vi "SingleMoleFinder.vi"(6 "Image Src":T1, 7 "error in":errorcluster, 18 "Min Radius (CircleDetection)":sgl=15.0, 19 "Max Radius (CircleDetection)":sgl=50.0, 21 "Keep/Remove Particles (Particle Filter 1)":bool=TRUE, 23 "Selection Values (Particle Filter 1)":T3(array[cluster])=[{"Measurement Parameter"=1, "Range Lower Value"=0.0, "Range Upper Value"=0.0, "Range"=FALSE, "Measurement Type"=FALSE}, {"Measurement Parameter"=0, "Range Lower Value"=15.0, "Range Upper Value"=100.0, "Range"=FALSE, "Measurement Type"=FALSE}] {"Measurement Parameter" items=["Center of Mass X", "Center of Mass Y", "First Pixel X", "First Pixel Y", "Bounding Rect Left", "Bounding Rect Top", "Bounding Rect Right", "Bounding Rect Bottom", "Max Feret Diameter Start X", "Max Feret Diameter Start Y", "Max Feret Diameter End X", "Max Feret Diameter End Y", "Max Horiz. Segment Length Left", "Max Horiz. Segment Length Right", "Max Horiz. Segment Length Row", "-", "Bounding Rect Width", "Bounding Rect Height", "Bounding Rect Diagonal", "Perimeter", "Convex Hull Perimeter", "Holes' Perimeter", "Max Feret Diameter", "Equivalent Ellipse Major Axis", "Equivalent Ellipse Minor Axis", "Equivalent Ellipse Minor Axis (Feret)", "Equivalent Rect Long Side", "Equivalent Rect Short Side", "Equivalent Rect Diagonal", "Equivalent Rect Short Side (Feret)", "Average Horiz. Segment Length", "Average Vert. Segment Length", "Hydraulic Radius", "Waddel Disk Diameter", "-", "Area", "Holes' Area", "Particle & Holes' Area", "Convex Hull Area", "Image Area", "-", "Number of Holes", "Number of Horiz. Segments", "Number of Vert. Segments", "-", "Orientation", "Max Feret Diameter Orientation", "-", "% Area/Image Area", "% Area/(Particle & Holes' Area)", "Ratio of Equivalent Ellipse Axes", "Ratio of Equivalent Rect Sides", "-", "Elongation Factor", "Compactness Factor", "Heywood Circularity Factor", "Type Factor", "-", "Sum X", "Sum Y", "Sum XX", "Sum XY", "Sum YY", "Sum XXX", "Sum XXY", "Sum XYY", "Sum YYY", "-", "Moment of Inertia XX", "Moment of Inertia XY", "Moment of Inertia YY", "Moment of Inertia XXX", "Moment of Inertia XXY", "Moment of Inertia XYY", "Moment of Inertia YYY", "Norm. Moment of Inertia XX", "Norm. Moment of Inertia XY", "Norm. Moment of Inertia YY", "Norm. Moment of Inertia XXX", "Norm. Moment of Inertia XXY", "Norm. Moment of Inertia XYY", "Norm. Moment of Inertia YYY", "Hu Moment 1", "Hu Moment 2", "Hu Moment 3", "Hu Moment 4", "Hu Moment 5", "Hu Moment 6", "Hu Moment 7"]}) -> (15 "Image Out":T1(plugin-control), 20 "Nb Circles (CircleDetection)":i32, 26 "Circles Data (CircleDetection)":T2(array[cluster]), 27 "error out":errorcluster)   [LabVIEW 2011]
uses:
  <vilib>/vision/Image Controls.llb/IMAQ Image.ctl
  <vilib>/vision/NI_Vision_Development_Module.lvlib
panel:
  out "Image Out 10":T1(plugin-control)
  out "Image Out 9":T1(plugin-control)
  out "Image Out 8":T1(plugin-control)
  out "Image Out 7":T1(plugin-control)
  out "Image Out 6":T1(plugin-control)
  out "Image Out 5":T1(plugin-control)
  out "Image Out 4":T1(plugin-control)
  out "Image Out 3":T1(plugin-control)
  out "Image Out 2":T1(plugin-control)
  out "Circles Data (calibrated)":T2(array[cluster])
  out "Number of Particles 2":i32
  out "Number of Particles":i32
  out "Particle Measurements (Pixels)":dbl[][](array[numeric]) format="%.2f"
  out "Particle Measurements (Real-World)":dbl[][](array[numeric]) format="%.2f"
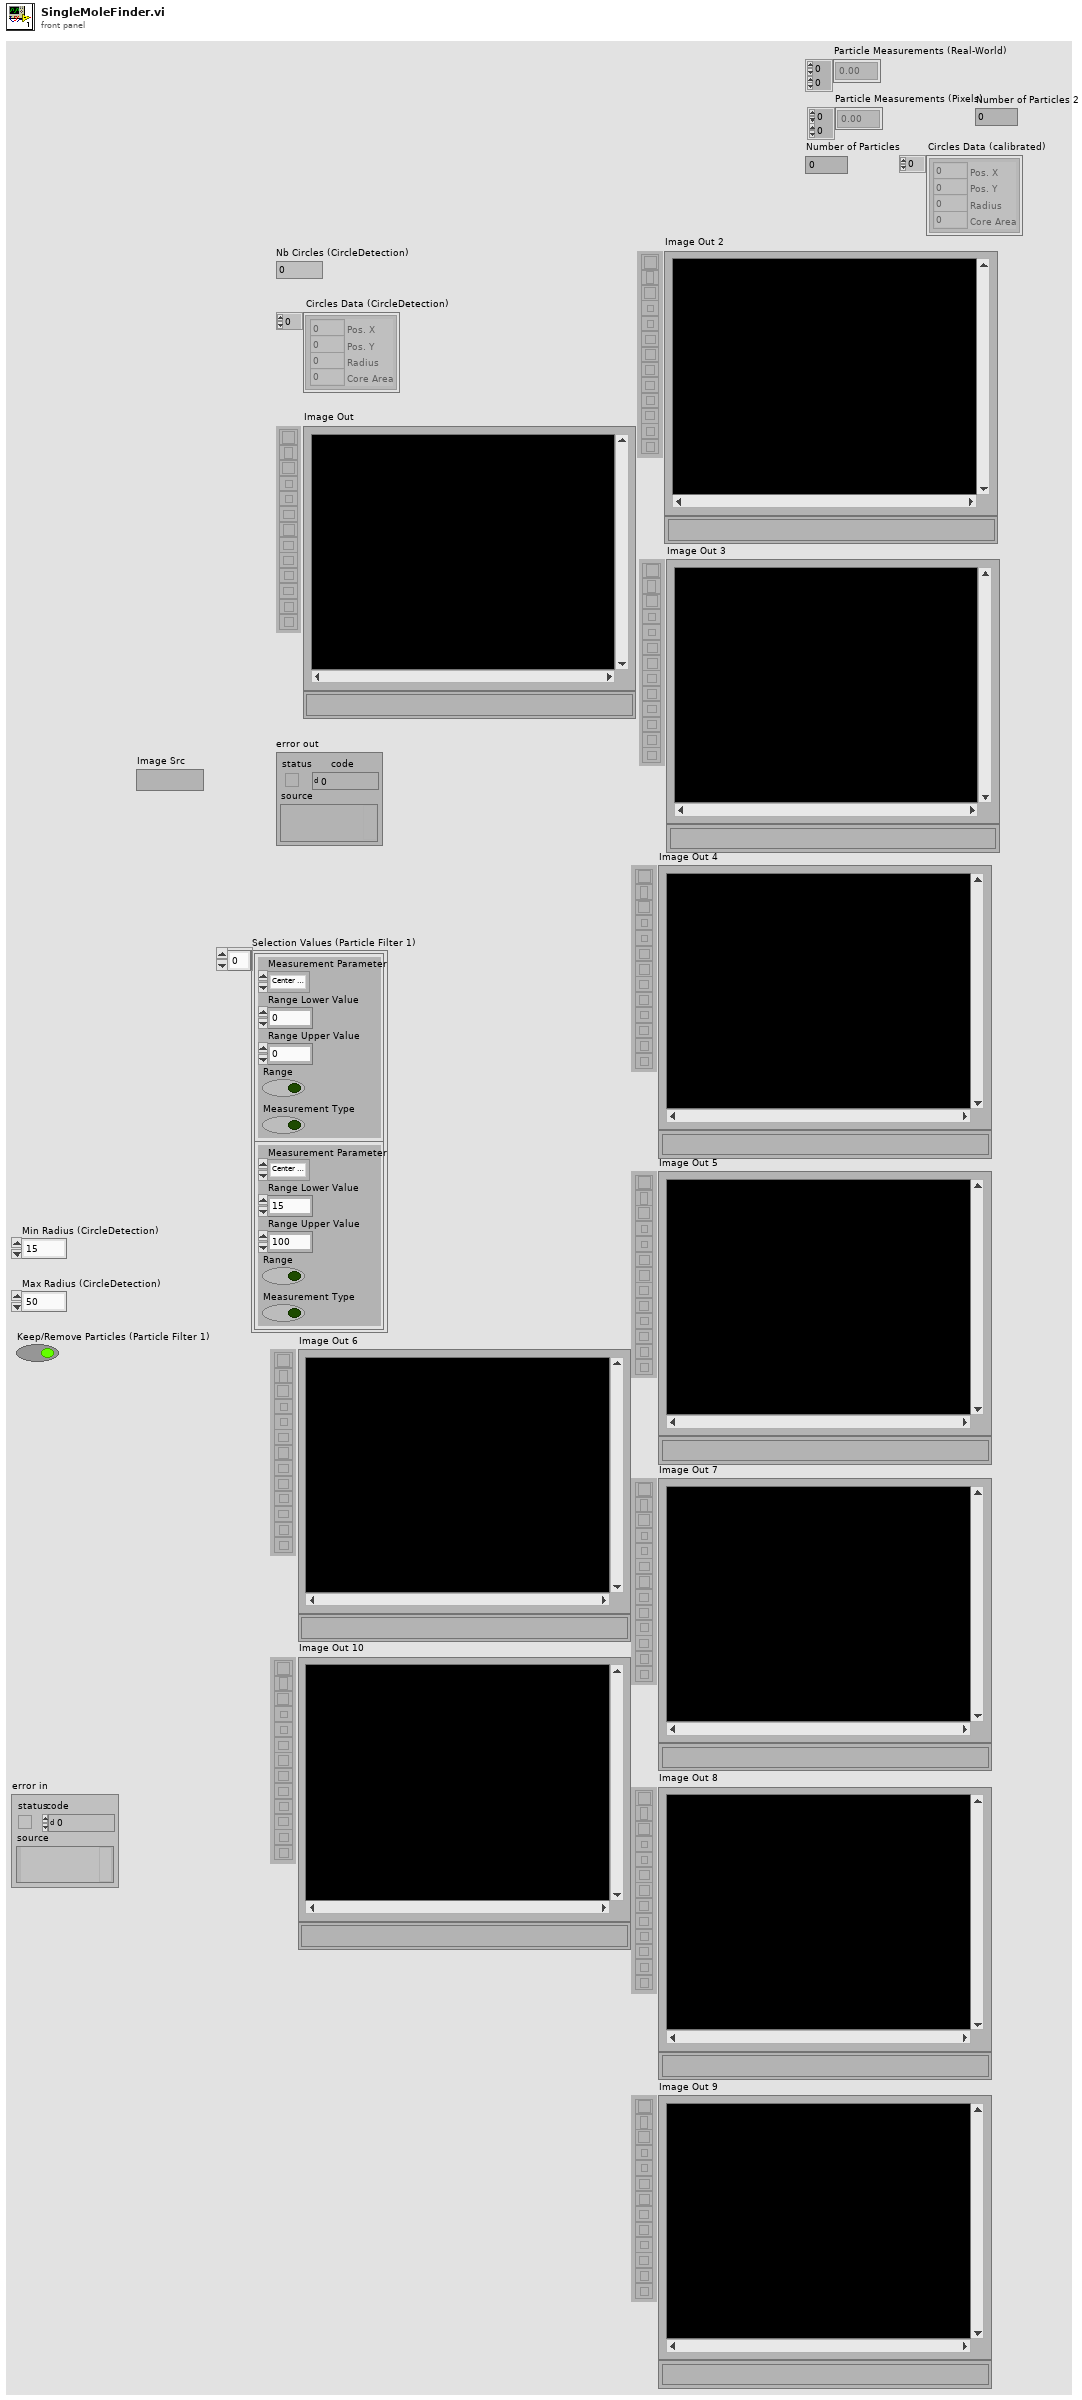
[diagram p1: front panel]
types:
  T1 = typedef "IMAQ Image.ctl" = refnum<image>
  T2 = cluster{"Pos. X":i32, "Pos. Y":i32, "Radius":i32, "Core Area":i32}[]
  T3 = cluster{"Measurement Parameter":i32, "Range Lower Value":dbl, "Range Upper Value":dbl, "Range":bool, "Measurement Type":bool}[]
  T4 = enum32{"AutoM", "Close", "Dilate", "Erode", "Gradient", "Gradient out", "Gradient in", "Hit miss", "Open", "PClose", "POpen", "Thick", "Thin"}
  T5 = enum32{"Linear", "Log", "Exp", "Square", "Square root", "Power X", "Power 1/X"}
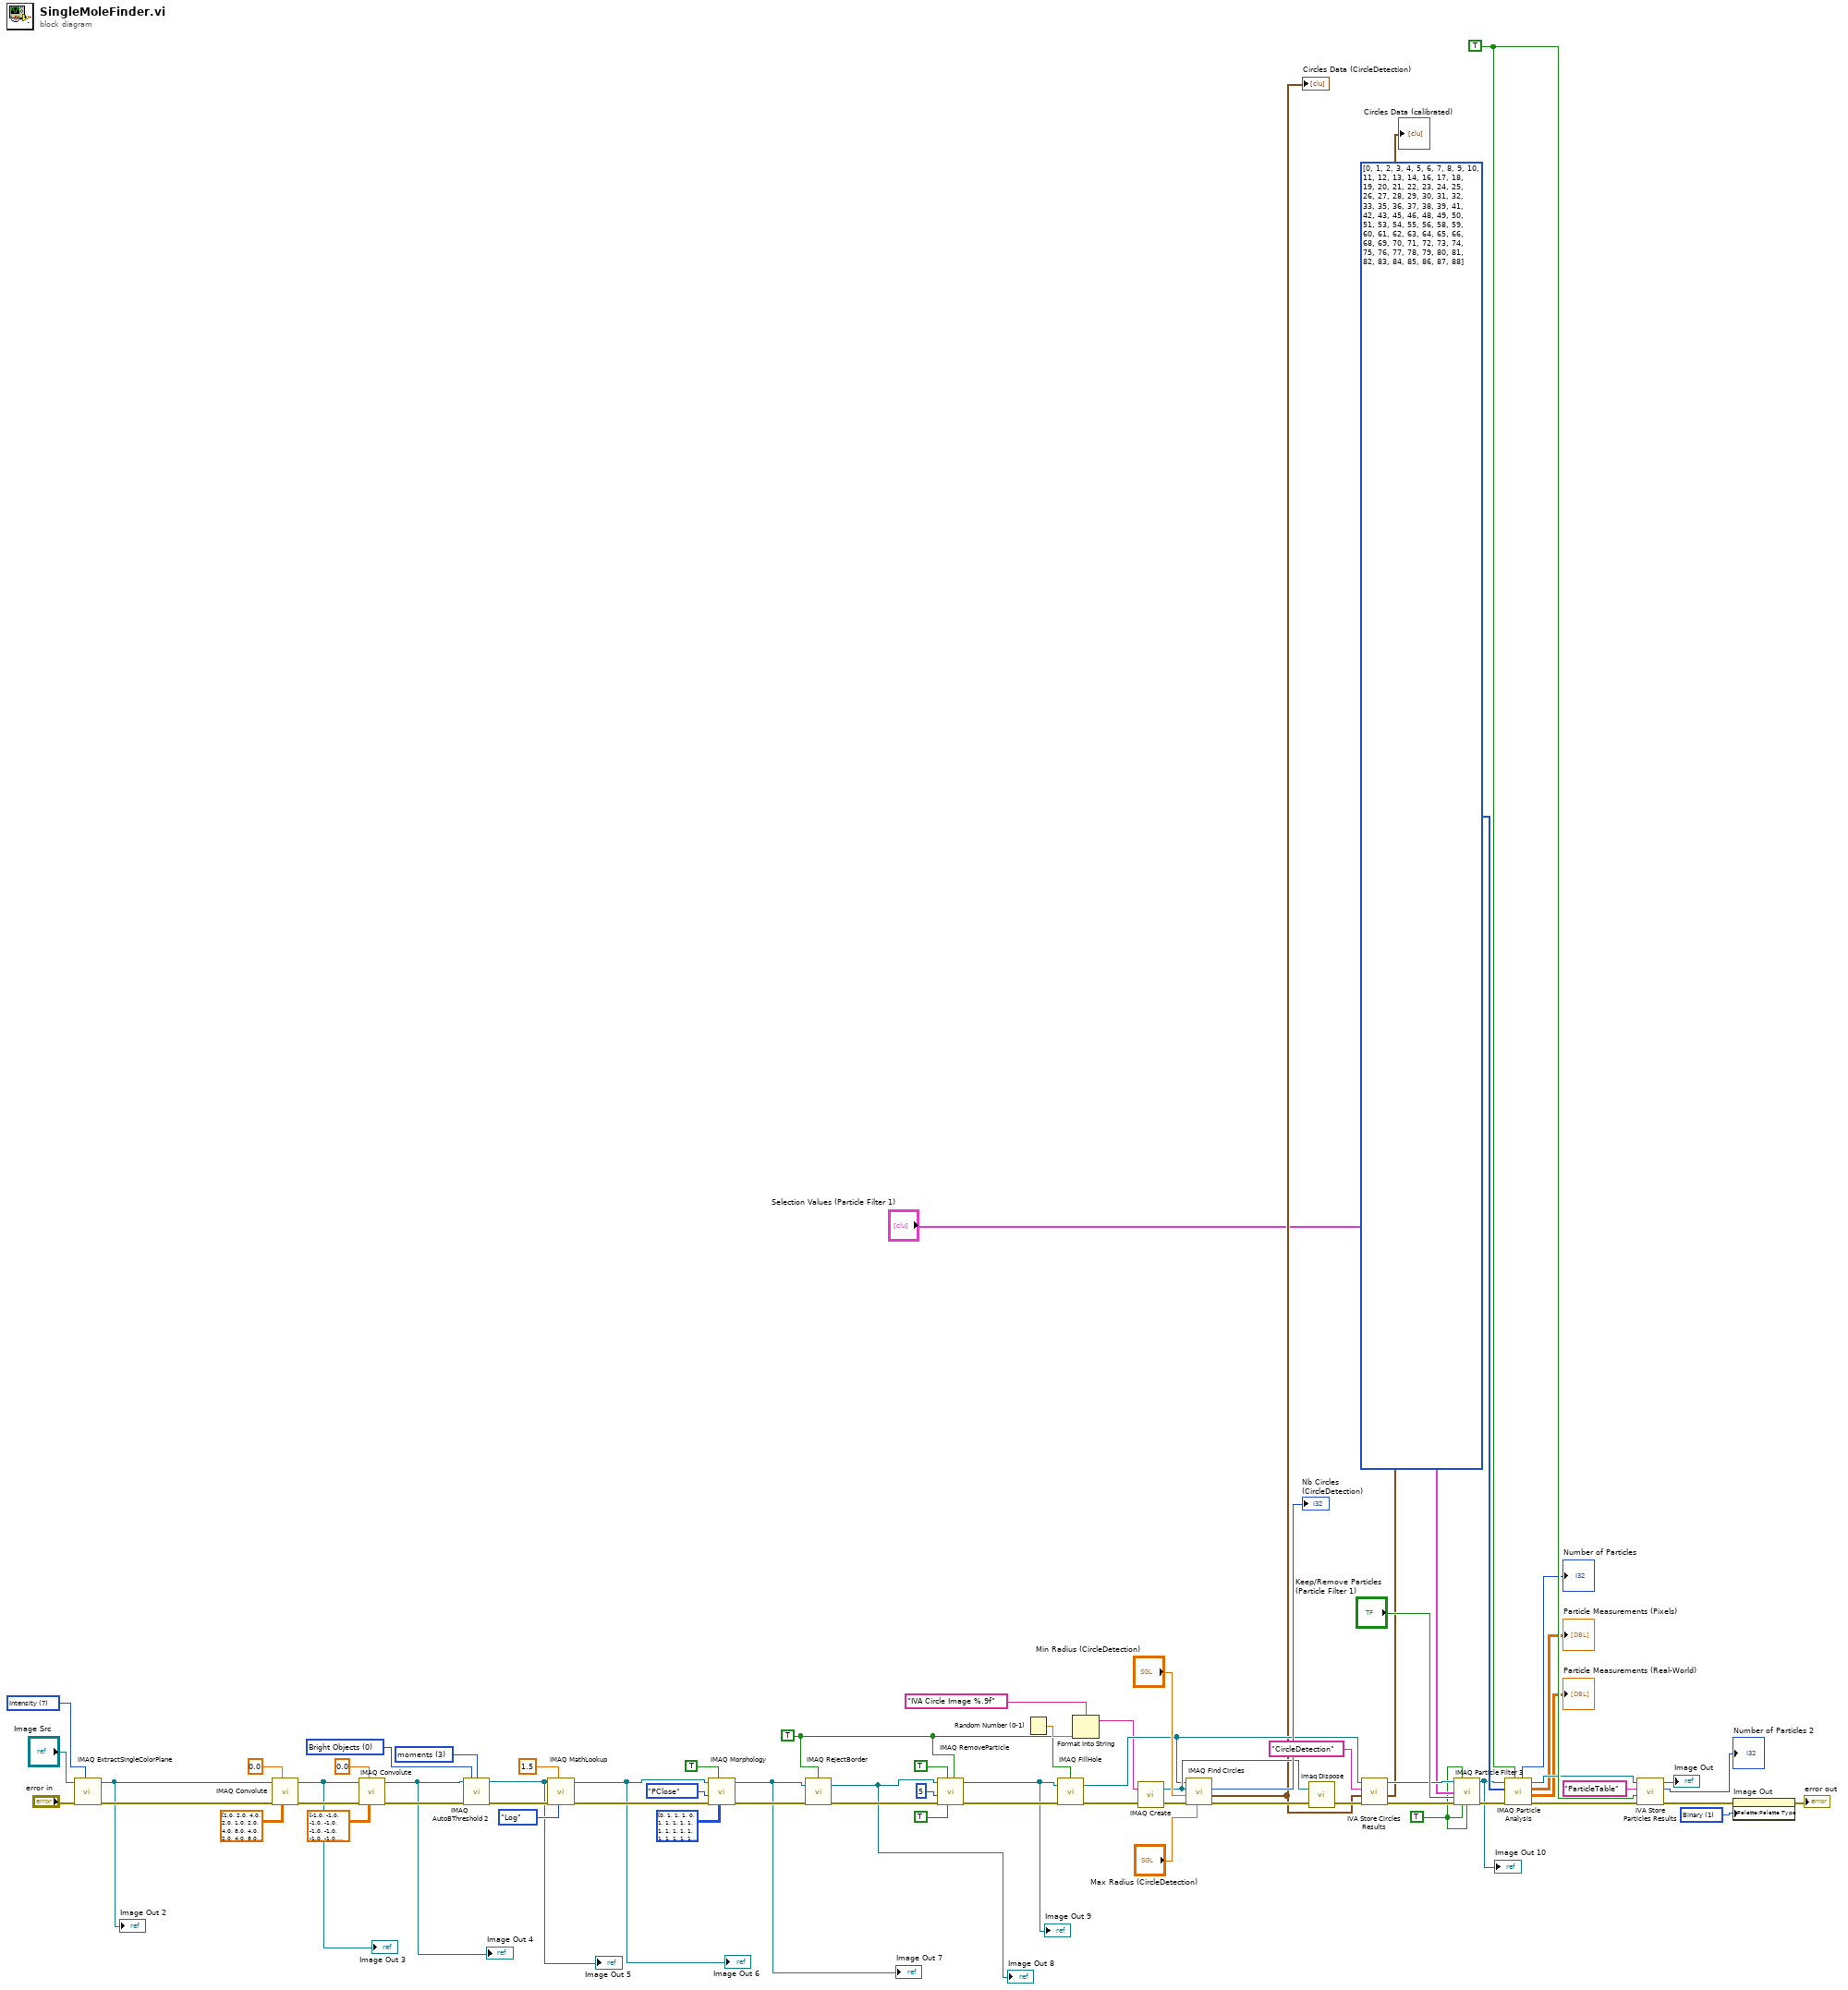
[diagram p0: block diagram]
diagram:
  w29 = i32[] [0, 1, 2, 3, 4, 5, 6, 7, 8, 9, 10, 11, 12, 13, 14, 16, 17, 18, 19, 20, 21, 22, 23, 24, 25, 26, 27, 28, 29, 30, 31, 32, 33, 35, 36, 37, 38, 39, 41, 42, 43, 45, 46, 48, 49, 50, 51, 53, 54, 55, 56, 58, 59, 60, 61, 62, 63, 64, 65, 66, 68, 69, 70, 71, 72, 73, 74, 75, 76, 77, 78, 79, 80, 81, 82, 83, 84, 85, 86, 87, 88] items=["Center of Mass X", "Center of Mass Y", "First Pixel X", "First Pixel Y", "Bounding Rect Left", "Bounding Rect Top", "Bounding Rect Right", "Bounding Rect Bottom", "Max Feret Diameter Start X", "Max Feret Diameter Start Y", "Max Feret Diameter End X", "Max Feret Diameter End Y", "Max Horiz. Segment Length Left", "Max Horiz. Segment Length Right", "Max Horiz. Segment Length Row", "-", "Bounding Rect Width", "Bounding Rect Height", "Bounding Rect Diagonal", "Perimeter", "Convex Hull Perimeter", "Holes' Perimeter", "Max Feret Diameter", "Equivalent Ellipse Major Axis", "Equivalent Ellipse Minor Axis", "Equivalent Ellipse Minor Axis (Feret)", "Equivalent Rect Long Side", "Equivalent Rect Short Side", "Equivalent Rect Diagonal", "Equivalent Rect Short Side (Feret)", "Average Horiz. Segment Length", "Average Vert. Segment Length", "Hydraulic Radius", "Waddel Disk Diameter", "-", "Area", "Holes' Area", "Particle & Holes' Area", "Convex Hull Area", "Image Area", "-", "Number of Holes", "Number of Horiz. Segments", "Number of Vert. Segments", "-", "Orientation", "Max Feret Diameter Orientation", "-", "% Area/Image Area", "% Area/(Particle & Holes' Area)", "Ratio of Equivalent Ellipse Axes", "Ratio of Equivalent Rect Sides", "-", "Elongation Factor", "Compactness Factor", "Heywood Circularity Factor", "Type Factor", "-", "Sum X", "Sum Y", "Sum XX", "Sum XY", "Sum YY", "Sum XXX", "Sum XXY", "Sum XYY", "Sum YYY", "-", "Moment of Inertia XX", "Moment of Inertia XY", "Moment of Inertia YY", "Moment of Inertia XXX", "Moment of Inertia XXY", "Moment of Inertia XYY", "Moment of Inertia YYY", "Norm. Moment of Inertia XX", "Norm. Moment of Inertia XY", "Norm. Moment of Inertia YY", "Norm. Moment of Inertia XXX", "Norm. Moment of Inertia XXY", "Norm. Moment of Inertia XYY", "Norm. Moment of Inertia YYY", "Hu Moment 1", "Hu Moment 2", "Hu Moment 3", "Hu Moment 4", "Hu Moment 5", "Hu Moment 6", "Hu Moment 7"] ("Pixel Measurements (ParticleTable)")
  w27 = TRUE ("Connectivity 4/8 (8) (ParticleTable)")
  w10 = TRUE ("Connectivity 4/8 (8) (Particle Filter 1)")
  w12 = TRUE ("Connectivity 4/8 (8) (FillHoles, RemoveBorderObjects and Remove Small Obkects)")
  w69 = 7 items=["Red", "Green", "Blue", "Hue", "Saturation", "Luminance", "Value", "Intensity"] ("Color Plane (IntensityExtraction)")
  w60 = 3 items=["clustering", "entropy", "metric", "moments", "inter-class variance"] ("Method (AutoTresholdMomentClustering)")
  w61 = u32 0 items=["Bright Objects", "Dark Objects"] ("Look For (AutoTresholdMomentClustering)")
  w22 = u32 1 items=["Grayscale", "Binary", "Gradient", "Rainbow", "Temperature", "User Defined"] ("Palette")
  n1 = call "IMAQ ExtractSingleColorPlane"("Color Plane"=w69, "error in (no error)"="error in", "Image Src"="Image Src") -> ("error out"=w67:errorcluster, "Image Dst Out"=w9:T1)  [unwired: 1 in, 6 out]
  "Image Out 2" <- w9
  n2 = call "IMAQ Convolute"("Kernel"=sgl[][] [[1.0, 2.0, 4.0, 2.0, 1.0], [2.0, 4.0, 8.0, 4.0, 2.0], [4.0, 8.0, 16.0, 8.0, 4.0], [2.0, 4.0, 8.0, 4.0, 2.0], [1.0, 2.0, 4.0, 2.0, 1.0]] ("Kernel (SmothingGaussian)"), "Divider (kernel sum)"=sgl 0.0 ("Divider (SmothingGaussian)"), "error in (no error)"=w67, "Image Src"=w9) -> ("error out"=w64:errorcluster, "Image Dst Out"=w8:T1)  [unwired: 3 in, 3 out]
  "Image Out 3" <- w8
  n3 = call "IMAQ Convolute"("Kernel"=sgl[][] [[-1.0, -1.0, -1.0, -1.0, -1.0], [-1.0, -1.0, -1.0, -1.0, -1.0], [-1.0, -1.0, 30.0, -1.0, -1.0], [-1.0, -1.0, -1.0, -1.0, -1.0], [-1.0, -1.0, -1.0, -1.0, -1.0]] ("Kernel (Convolution)"), "Divider (kernel sum)"=sgl 0.0 ("Divider (Convolution)"), "error in (no error)"=w64, "Image Src"=w8) -> ("error out"=w62:errorcluster, "Image Dst Out"=w7:T1)  [unwired: 3 in, 3 out]
  "Image Out 4" <- w7
  n4 = call "IMAQ AutoBThreshold 2"("Image Src"=w7, "Look For (Bright Objects)"=w61, "Method (clustering)"=w60, "error in (no error)"=w62) -> ("Image Dst Out"=w6:T1, "error out"=w57:errorcluster)  [unwired: 4 in, 6 out]
  "Image Out 5" <- w6
  n5 = call "IMAQ MathLookup"("Operator"=T5."Log" ("Operator (LogarithmicSmoother)"), "X Value"=sgl 1.5 ("X Value (LogarithmicSmoother)"), "error in (no error)"=w57, "Image Src"=w6) -> ("error out"=w53:errorcluster, "Image Dst Out"=w5:T1)  [unwired: 3 in, 3 out]
  "Image Out 6" <- w5
  n6 = call "IMAQ Morphology"("Structuring Element"=i32[][] [[0, 1, 1, 1, 0], [1, 1, 1, 1, 1], [1, 1, 1, 1, 1], [1, 1, 1, 1, 1], [0, 1, 1, 1, 0]] ("Structuring Element (closeObjects)"), "Square/Hexa (Square)"=TRUE ("Square/Hexa (Square) (closeObjects)"), "error in (no error)"=w53, "Operation"=T4."PClose" ("Operation (closeObjects)"), "Image Src"=w5) -> ("error out"=w52:errorcluster, "Image Dst Out"=w4:T1)  [unwired: 2 in, 3 out]
  "Image Out 7" <- w4
  n7 = call "IMAQ RejectBorder"("error in (no error)"=w52, "Image Src"=w4, "Connectivity 4/8 (8)"=w12) -> ("error out"=w49:errorcluster, "Image Dst Out"=w3:T1)  [unwired: 1 in, 2 out]
  "Image Out 8" <- w3
  n8 = call "IMAQ RemoveParticle"("Connectivity 4/8 (8)"=w12, "Low Pass/High Pass (Low)"=TRUE ("Low Pass/High Pass (Low) (RemoveSmallObjects)"), "Square/Hexa (Square)"=TRUE ("Square/Hexa (Square) (RemoveSmallObjects)"), "error in (no error)"=w49, "Number of Erosion"=5, "Image Src"=w3) -> ("error out"=w48:errorcluster, "Image Dst Out"=w2:T1)  [unwired: 1 in, 3 out]
  "Image Out 9" <- w2
  n9 = Random Number (0-1)() -> (number: 0 to 1=w34:dbl)
  n10 = call "IMAQ FillHole"("error in (no error)"=w48, "Image Src"=w2, "Connectivity 4/8 (8)"=w12) -> ("error out"=w42:errorcluster, "Image Dst Out"=w39:T1)  [unwired: 1 in, 2 out]
  n11 = Format Into String(format string="IVA Circle Image %.9f" ("Image Name"), w34) -> (resulting string=w36:string)  [unwired: 2 in, 1 out]
  n12 = call "IMAQ Create"("Image Name"=w36, "error in (no error)"=w42) -> ("New Image"=w44:T1, "error out"=w43:errorcluster)  [unwired: 2 in, 1 out]
  n13 = call "IMAQ Find Circles"("Max Radius"="Max Radius (CircleDetection)", "error in (no error)"=w43, "Min Radius"="Min Radius (CircleDetection)", "Image Dst"=w44, "Image Src"=w39) -> ("error out"=w41:errorcluster, "Circles Data"=w37:T2, "Nb Circles"=→"Nb Circles (CircleDetection)":i32)  [unwired: 4 out]
  "Circles Data (CircleDetection)" <- w37
  n14 = call "Imaq Dispose"("Image"=w44, "error in (no error)"=w41) -> ("error out"=w40:errorcluster)  [unwired: 1 in, 3 out]
  n15 = call <vilib>:"IVA Store Circles Results.vi"("error in (no error)"=w40, "Circles Data"=w37, "Step Name"="CircleDetection", "Image in"=w39) -> ("error out"=w31:errorcluster, "Circles Data (calibrated)"=→"Circles Data (calibrated)":T2, "Image dup"=w32:T1)  [unwired: 5 out]
  n16 = call "IMAQ Particle Filter 3"("Image Src"=w32, "Connectivity 4/8 (8)"=w10, "Selection Values"="Selection Values (Particle Filter 1)", "Keep/Remove Particles (F)"="Keep/Remove Particles (Particle Filter 1)", "error in (no error)"=w31, "Reject Border? (F)"=w10, "Fill Holes? (F)"=w10) -> ("Image Dst Out"=w1:T1, "error out"=w28:errorcluster)  [unwired: 2 in, 5 out]
  "Image Out 10" <- w1
  n17 = call "IMAQ Particle Analysis"("Connectivity 4/8 (8)"=w27, "error in (no error)"=w28, "Pixel Measurements"=w29, "Image"=w1) -> ("error out"=w24:errorcluster, "Particle Measurements (Real-World)"=→"Particle Measurements (Real-World)":dbl[][], "Particle Measurements (Pixels)"=→"Particle Measurements (Pixels)":dbl[][], "Image Out (duplicate)"=w26:T1, "Number of Particles"=→"Number of Particles":i32)  [unwired: 1 in, 2 out]
  n18 = call <vilib>:"IVA Store Particles Results.vi"("error in (no error)"=w24, "Connectivity 4/8 (8)"=w27, "Step Name"="ParticleTable", "Image in"=w26) -> ("error out"=w21:errorcluster, "Number of Particles"=→"Number of Particles 2":i32, "Image dup"=→"Image Out":T1)  [unwired: 5 out]
  n19 = property on="Image Out" class="ImageControl"(error in=w21, "Palette:Palette Type"=w22) -> (error out=→"error out":errorcluster)  [unwired: 1 in, 1 out]
